vi "Tx Generic.vi"(8 "error in (no error)":errorcluster, 11 "Node Ptr":T3 format="%.0x") -> (0 "error out":errorcluster)   [LabVIEW 2020, in "AIM ARINC 664 System Explorer.lvlib" / "Implementation.lvlib"]
uses:
  Implementation.lvlib
  <vilib>/NI VeriStand/Custom Device API/Custom Device Item Ref.ctl
  Shared/RawFrame_entry.ctl
  <instrlib>/AIM GmbH/_AIM 664/_controls/queue_header_generic.ctl
  <vilib>/NI VeriStand/Custom Device API/Custom Device API.lvlib
  Scripting/AIM ARINC 664 Scripting.lvlib
  <instrlib>/AIM GmbH/_AIM 664/AIM664LV.lvlib
panel:
  in  "Frame List":i32(listbox)
  in  "SHDocVw.IWebBrowser":refnum<k7>(container)
  out "Number of Frames":i32
  out "Frame Configurations":T1[](array[typedef]) {"HeaderInfo"."NetSelect" items=["FDX_TX_FRAME_DLY_A"=0, "FDX_TX_FRAME_DLY_B"=1, "FDX_TX_FRAME_BOTH "=3, "FDX_TX_FRAME_ONLY_A"=4, "FDX_TX_FRAME_ONLY_B "=5]; "HeaderInfo"."FrameStartMode" items=["FDX_TX_FRAME_START_IFG", "FDX_TX_FRAME_START_PGWT", "FDX_TX_FRAME_START_TRG"]; "HeaderInfo"."PhysErrorInjection" items=["FDX_TX_FRAME_ERR_OFF"=0, "FDX_TX_FRAME_ERR_CRC"=1, "FDX_TX_FRAME_ERR_ALI"=2, "FDX_TX_FRAME_ERR_PRE"=4, "FDX_TX_FRAME_ERR_PHY"=8]; "HeaderInfo"."SequenceNumberInit" items=["FDX_TX_FRAME_SEQ_INIT_AUTO"=65535]; "HeaderInfo"."SequenceNumberOffset" items=["FDX_TX_FRAME_SEQ_OFFS_AUTO "=65535]; "HeaderInfo"."PayloadGenerationMode" items=["FDX_TX_FRAME_PGM_USER"=0, "FDX_TX_FRAME_PGM_IP_PART"=1, "FDX_TX_FRAME_PGM_IP_FULL"=2, "FDX_TX_FRAME_PGM_IP_PART_TT"=10, "FDX_TX_FRAME_PGM_IP_FULL_TT"=20]; "HeaderInfo"."PayloadBufferMode" items=["FDX_TX_FRAME_PBM_STD", "FDX_TX_FRAME_PBM_MAC", "FDX_TX_FRAME_PBM_UDP"]}
  out "Name":string
  in  "Property List":i32(listbox)
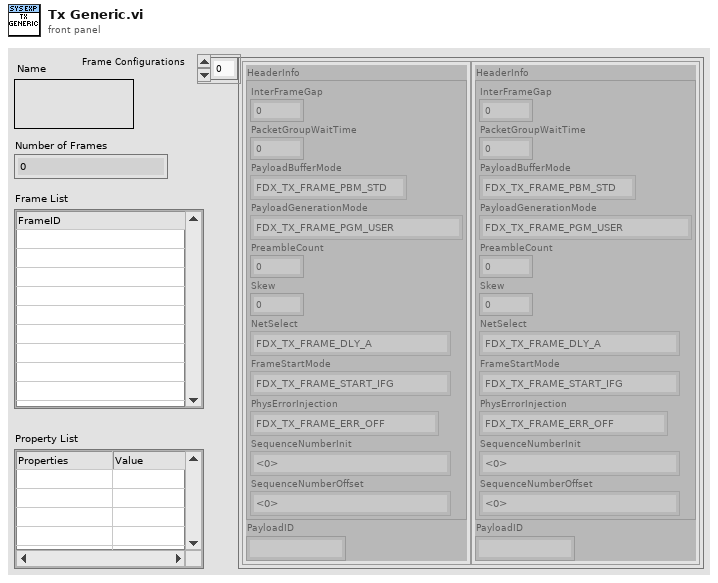
[diagram p1: front panel]
types:
  T1 = typedef "RawFrame_entry.ctl" = cluster{"HeaderInfo":T2, "PayloadID":string}
  T2 = typedef "AIM664LV.lvlib/queue_header_generic.ctl" = cluster{"InterFrameGap":u32, "PacketGroupWaitTime":u32, "PayloadBufferMode":u8, "PayloadGenerationMode":u8, "PreambleCount":u8, "Skew":u32, "NetSelect":u8, "FrameStartMode":u8, "PhysErrorInjection":u32, "SequenceNumberInit":u16, "SequenceNumberOffset":u16}
  T3 = typedef "Custom Device API.lvlib/Custom Device Item Ref.ctl" = u64
  T4 = typedef "Custom Device API.lvlib/Custom Device Item Info.ctl" = cluster{"Name":string, "Is Channel":bool, "GUID":string, "Is Waveform":bool}
  T5 = typedef "Custom Device API.lvlib/Custom Device Commands.ctl" = enum16{"Default", "Item renamed", "Shutdown", "Dynamic button pressed"}
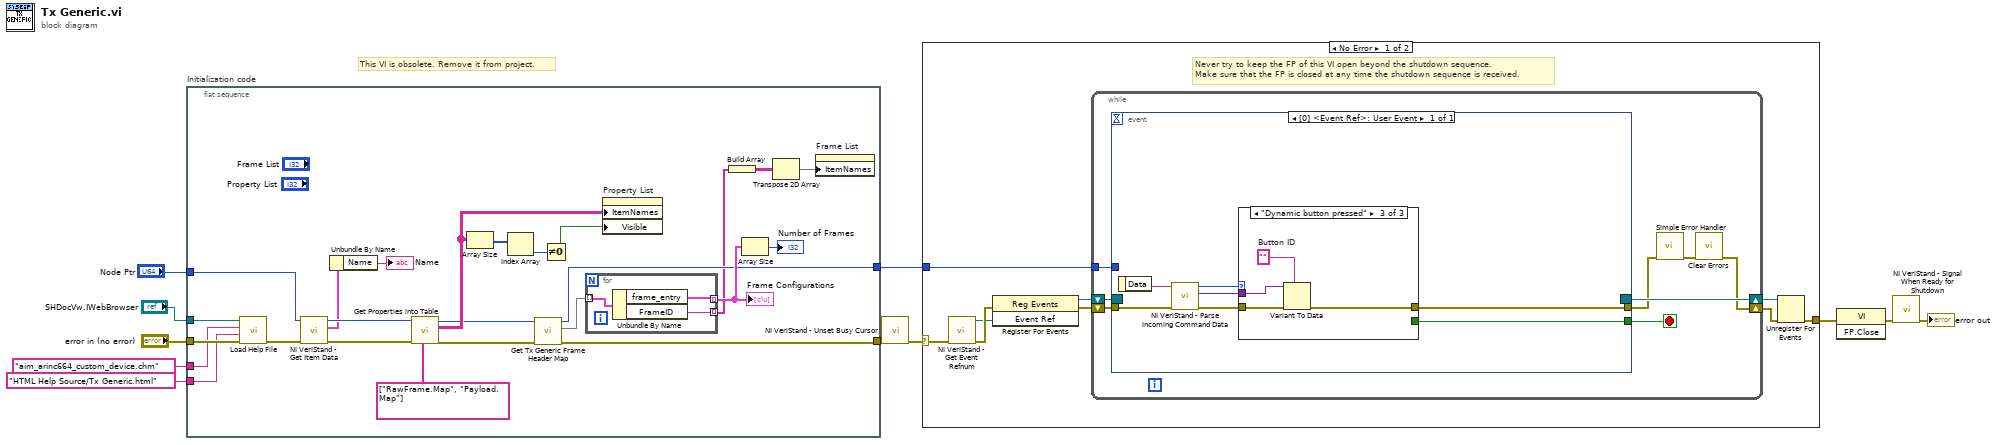
[diagram p0: block diagram]
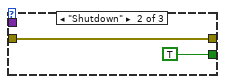
[diagram p3: hidden frame]
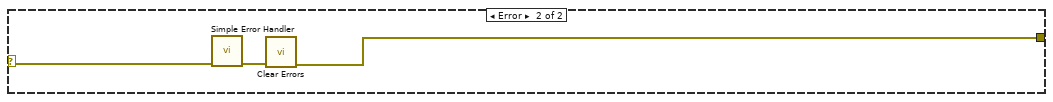
[diagram p4: hidden frame]
diagram:
  # "This VI is obsolete. Remove it from project."
  n1 = flat-sequence "Initialization code" {
    tunnel: "error in (no error)" -> [w24]
    tunnel: "Node Ptr" -> [w27]
    tunnel: [w17] -> w5
    tunnel: [w16] -> w4
    tunnel: "SHDocVw.IWebBrowser" -> [w22]
    tunnel: "aim_arinc664_custom_device.chm" ("CD_CHM_FileName") -> [w21]
    tunnel: "HTML Help Source/Tx Generic.html" ("CD_CHM_Section") -> [w20]
    frame #0 {
      n2 = call "Load Help File.vi"("error in (no error)"=w24, "HTML File to Load"=w20, "Main CHM File"=w21, "Browser"=w22) -> ("error out"=w23:errorcluster)  [unwired: 6 in, 1 out]
      n3 = call <vilib>:"NI VeriStand - Get Item Data.vi"("error in (no error)"=w23, "Item Ref in"=w27) -> ("error out"=w28:errorcluster, "Item Info"=w35:T4, "Item Ref out"=w36:T3)  [unwired: 7 out]
      n4 = Unbundle By Name(w35) -> ("Name"=→"Name":string)
      n5 = call "Get Properties into Table.vi"("Blacklisted properites"=string[] ["RawFrame.Map", "Payload.Map"], "error in"=w28, "Item Ref in"=w36) -> ("error out"=w18:errorcluster, "Property Names"=w32:string[][], "Item Ref out"=w19:T3)  [unwired: 6 in]
      n6 = Array Size(array=w32) -> (size(s)=w33:i32[])
      n7 = Index Array(array=w33) -> (element=w34:i32)  [unwired: 1 in]
      n8 = call "Get Tx Generic Frame Header Map.vi"("error in"=w18, "custom device ref in"=w19) -> ("error out"=w16:errorcluster, "Raw Frame Header Map"=w15:map{string, T1}, "custom device ref out"=w17:T3)  [unwired: 7 in]
      n9 = Not Equal To 0?(x=w34) -> (x != 0?=w31:bool)
      n10 = for {
        tunnel: w15 -> [w39] mode=indexing
        tunnel: [w38] -> w25 mode=indexing
        tunnel: [w37] -> w14 mode=indexing
        n11 = Unbundle By Name(w39) -> ("frame_entry"=w38:T1, "FrameID"=w37:string)
      }
      "Frame Configurations" <- w25
      n12 = property on="Property List" class="MCListbox (strict)"("ItemNames"=w32, "Visible"=w31) -> ()  [unwired: 2 in, 2 out]
      n13 = Build Array(w14) -> (w13:string[][])
      n14 = Array Size(array=w25) -> (size(s)=→"Number of Frames":i32)
      n15 = Transpose 2D Array(2D array=w13) -> (transposed array=w12:string[][])
      n16 = property on="Frame List" class="MCListbox (strict)"("ItemNames"=w12) -> ()  [unwired: 2 in, 2 out]
    }
  }
  n17 = call <vilib>:"NI VeriStand - Unset Busy Cursor.vi"("error in (no error)"=w4) -> ("error out"=w7:errorcluster)  [unwired: 10 out]
  n18 = case shown="No Error" w7 {
    selector: w7 -> [w41 w73]
    tunnel: [w45 w71] -> w11
    tunnel: w5 -> [w40 _]
    frame No Error {
      # "Never try to keep the FP of this VI open beyond the shutdown sequence.\nMake sure that the FP is closed at any time the shutdown sequence is received."
      n19 = call <vilib>:"NI VeriStand - Get Event Refnum.vi"("error in (no error)"=w41) -> ("error out"=w48:errorcluster, "Event Ref"=w44:refnum<user-event>)  [unwired: 9 out]
      n20 = register-events(error in=w48, w44) -> (reference out=w42:refnum<event-registration>, error out=w43:errorcluster)  [unwired: 1 in]
      n21 = while {
        shift-right: [w50] -> w46
        shift-left: w43 -> [w55]
        shift-right: [w56] -> w47
        shift-left: w42 -> [w54]
        tunnel: w40 -> [w49]
        stop <- w53 stop-if-true
        n22 = event shown="[0] <Event Ref>: User Event" {
          selector: w54 -> [_]
          dyn-events: [_] -> w56
          timeout: _ -> [_]
          tunnel: w55 -> [w63]
          tunnel: [w59] -> w53
          tunnel: [w58] -> w52
          tunnel: w49 -> [_]
          event User Event {
            n23 = event-data() -> ("Data"=w62:string)  [unwired: 1 out]
            n24 = call <vilib>:"NI VeriStand - Parse Incoming Command Data.vi"("error in (no error)"=w63, "Incoming data"=w62) -> ("error out"=w61:errorcluster, "Outgoing data"=w57:variant, "Action"=w60:T5)  [unwired: 7 out]
            n25 = case shown="\"Dynamic button pressed\"" w60 {
              tunnel: w61 -> [w64 w65 w70]
              tunnel: [_ TRUE _] -> w59
              tunnel: [w64 w65 w67] -> w58
              tunnel: w57 -> [_ _ w69]
              frame "Default", Default {
              }
              frame "Shutdown" {
              }
              frame "Dynamic button pressed" {
                w68 = ""  # Button ID
                n26 = Variant To Data(error in=w70, type=w68, Variant=w69) -> (error out=w67:errorcluster)  [unwired: 1 out]
              }
            }
          }
        }
        n27 = call <vilib>:"Simple Error Handler.vi"("error in (no error)"=w52) -> ("error out"=w51:errorcluster)  [unwired: 1 in, 7 out]
        n28 = call <vilib>:"Clear Errors.vi"("error in (no error)"=w51) -> ("error out"=w50:errorcluster)  [unwired: 1 in, 5 out]
      }
      n29 = Unregister For Events(event registration refnum=w47, error in=w46) -> (error out=w45:errorcluster)
    }
    frame Error {
      n30 = call <vilib>:"Simple Error Handler.vi"("error in (no error)"=w73) -> ("error out"=w72:errorcluster)  [unwired: 1 in, 7 out]
      n31 = call <vilib>:"Clear Errors.vi"("error in (no error)"=w72) -> ("error out"=w71:errorcluster)  [unwired: 1 in, 5 out]
    }
  }
  n32 = invoke class="VI" method="FP.Close"(error in=w11) -> (error out=w10:errorcluster)  [unwired: 2 in, 2 out]
  n33 = call <vilib>:"NI VeriStand - Signal When Ready for Shutdown.vi"("error in (no error)"=w10) -> ("error out"=→"error out":errorcluster)  [unwired: 10 out]
